vi "parse_digital_io_command.vi"(4 "error in":errorcluster, 7 "msg in":string) -> (0 "error out":errorcluster, 2 "digital IO":cluster{"name":string, "value":bool}, 3 "msg out":string)   [LabVIEW 2015]
doc: "Parses a message into a digital IO command"
uses:
  std_msgs/subs/parse_string_scalar.vi
  std_msgs/subs/parse_bool_scalar.vi
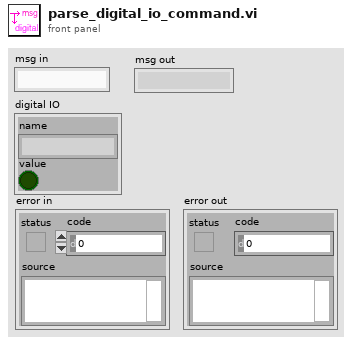
[diagram p1: front panel]
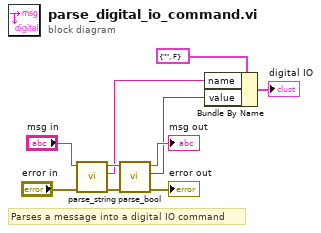
[diagram p0: block diagram]
diagram:
  # "Parses a message into a digital IO command"
  n1 = call-poly "parse_string.vi"("error in"="error in", "msg in"="msg in") -> ("error out"=w8:errorcluster, "string"=w3:string, "msg out"=w7:string)  [unwired: 3 in]
  n2 = call-poly "parse_bool.vi"("error in"=w8, "msg in"=w7) -> ("error out"=→"error out":errorcluster, "bool"=w2:bool, "msg out"=→"msg out":string)  [unwired: 3 in]
  n3 = Bundle By Name(cluster=cluster{"name":string, "value":bool} {"name"="", "value"=FALSE}, "name"=w3, "value"=w2) -> (→"digital IO":cluster{"name":string, "value":bool})
